vi "UI.vi"(0 "reference in":refnum<class "GUI NVM.lvclass">, 5 "error in (no error)":errorcluster) -> (14 "reference out":refnum<class "GUI NVM.lvclass">, 19 "error out":errorcluster)   [LabVIEW 2019, in "GUI NVM.lvclass"]
uses:
  GUI NVM.lvclass
  D:/GIT H4000/H4000/src/GUI_class/GUI.lvclass
  modbus engine custom/MB_ENGINE_class/Engine Alarms.ctl
  modbus engine custom/MB_ENGINE_class/Settings.ctl
  modbus engine custom/MB_ENGINE_class/cmd enum.ctl
  modbus engine custom/MB_ENGINE_class/Engine State.ctl
  GUI_class/GUI.lvclass/GUI.ctl
  TypeDef/Needle Valve Data.ctl
  TypeDef/Needle Valve State.ctl
  modbus engine custom/MB_ENGINE_class/Limits Status.ctl
  SV_Wrap/SharedVariableWrapper.lvclass/SharedVariableWrapper.ctl
  MessageAMC_class/MessageAMC.lvclass
  D:/GIT H4000/H4000/src/MessageInterface_class/MessageInterface.lvclass
  TypeDef/Needle Valve Settings.ctl
  0872259c-c1b7-4622-8eff-96544e628326.vi
  1b4fed76-272f-4eb9-b435-1b7916789d73.vi
  d0ca9bf2-7cd9-4c29-a03d-de1c10393a74.vi
  GUI_class/Set Win State.vi
  GUI_class/protected/GetSheredData.vi
  0872259c-c1b7-4622-8eff-96544e628326.vi/63923c93-3271-404a-8daf-727763f159bc.vi
  SV_Wrap/Write Var Info.vi
  SV_Wrap/Read Var Info.vi
  1b4fed76-272f-4eb9-b435-1b7916789d73.vi/fad6aa2d-1fd6-40e9-9208-cebdd25b163b.vi
  d0ca9bf2-7cd9-4c29-a03d-de1c10393a74.vi/ea186c4c-0445-4979-bfc0-5907181f2b8f.vi
  SV_Wrap/Read connection str.vi
  <userlib>/_OpenG.lib/time/time.llb/Tick Count (ms)__ogtk.vi
  GUI_class/GUI.lvclass
  MessageInterface_class/MessageInterface.lvclass
  SV_Wrap/SharedVariableWrapper.lvclass
  modbus engine custom/MB_ENGINE_class/MB_ENGINE.lvclass
panel:
  in  "Engine State":T1 items=["ACCELERATING", "DECELERATINGTOSTOP", "DECELERATING", "STEADY", "INDEX_ACCEL", "NDEX_RUN", "INDEX_DECEL", "INDEX_DWELL", "INACTIVE", "STANDBY", "STANDBYTOINACTIVE"]
  out "String 2":string
  out "String":string
  in  "clear fault":bool
  in  "stop":bool
  in  "close":bool
  in  "open":bool
  in  "Set_cmd":bool
  in  "cmd to write":T2 items=["0 Idle"=0, "1 GoTo Absolute Position"=1, "2 GoTo Relative"=2, "10 GoTo Home Position"=10, "11 Set Home Position"=11, "12 Set FindHome Mode"=12, "13 Reset FindHome Mode"=13, "14 Get FindHome State"=14, "20 Hard Stop"=20, "21 HiZ Stop"=21, "22 Soft Stop"=22, "30 Clear Fault"=30, "40 Encoder Set Home"=40, "70 Driver Init"=70]
  in  "set":bool
  out "Kinematic":T3
  out "Waveform Chart - Dark 3":dbl(graph) caption="Угол"
  out "encoder":i32(graph) caption="Энкодер"
  out "step":i32(graph) caption="ШАГ"
  out "Alarms":T4
  out "DO 19":bool
  out "Connect":bool
  in  "stop":bool
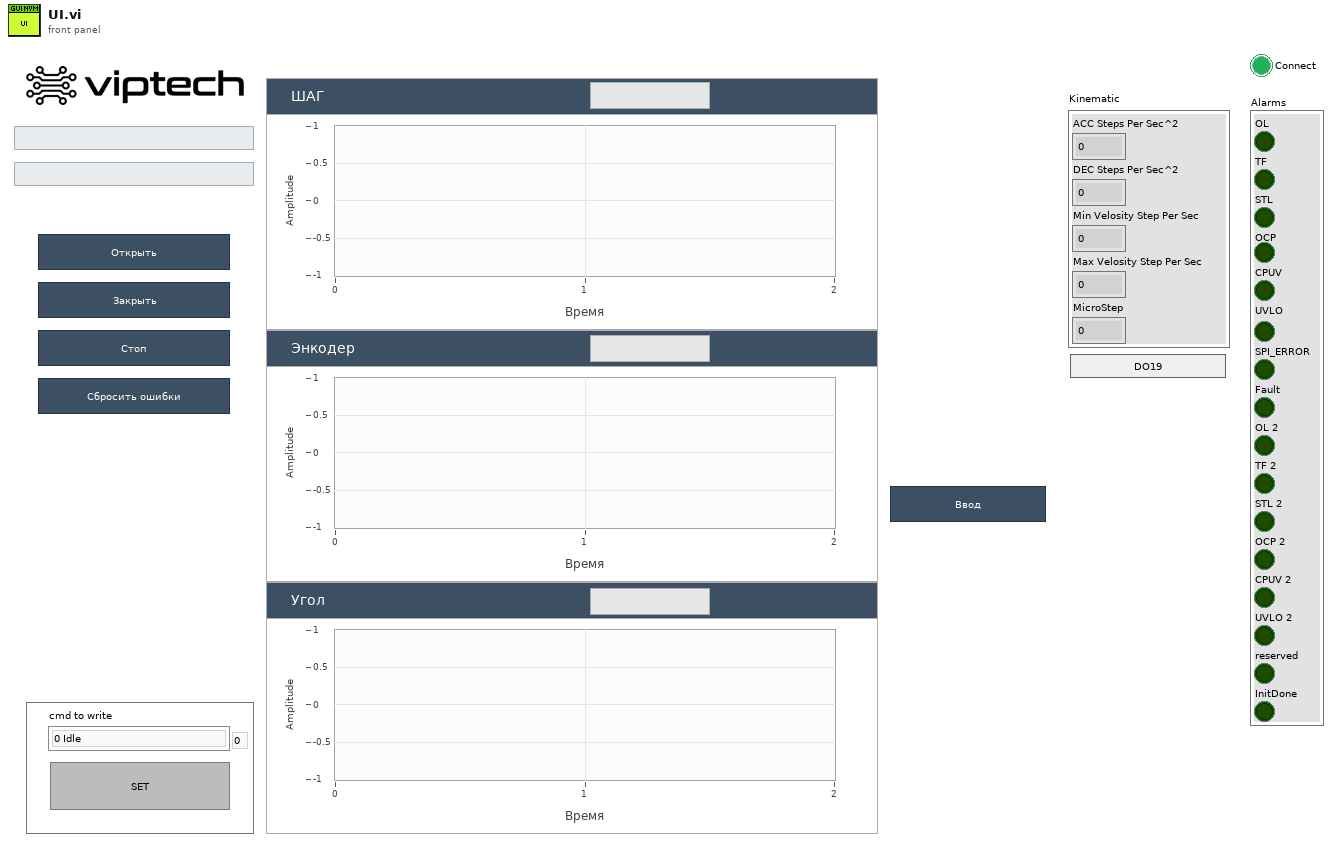
[diagram p1: front panel]
types:
  T1 = typedef "MB_ENGINE.lvclass/Engine State.ctl" = u16
  T2 = typedef "MB_ENGINE.lvclass/cmd enum.ctl" = u16
  T3 = typedef "MB_ENGINE.lvclass/Settings.ctl" = cluster{"ACC Steps Per Sec^2":u16, "DEC Steps Per Sec^2":u16, "Min Velosity Step Per Sec":u16, "Max Velosity Step Per Sec":u16, "MicroStep":u16}
  T4 = typedef "MB_ENGINE.lvclass/Engine Alarms.ctl" = cluster{"OL":bool, "TF":bool, "STL":bool, "OCP":bool, "CPUV":bool, "UVLO":bool, "SPI_ERROR":bool, "Fault":bool, "OL 2":bool, "TF 2":bool, "STL 2":bool, "OCP 2":bool, "CPUV 2":bool, "UVLO 2":bool, "reserved":bool, "InitDone":bool}
  T5 = enum32{"Invalid", "Standard", "Closed", "Hidden", "Minimized", "Maximized"}
  T6 = enum32{"invalid app kind", "Development System", "Run Time System", "Student Edition", "Embedded LabVIEW", "Evaluation", "Custom"}
  T7 = typedef "Needle Valve Settings.ctl" = cluster{"average size":i32, "open force":u16, "close force":u16, "open settings":T3, "close settings":T3}
  T8 = typedef "SharedVariableWrapper.lvclass/Config.ctl" = cluster{"connection str":string, "timeout":dbl, "ip":string}
  T9 = cluster{"Core":cluster{"Current VI Reference":refnum<vi>, "Close Panel on Exit?":bool}, "amc":refnum<class "MessageAMC.lvclass">, "settings_name_1":string}
  T10 = cluster{"Current VI Reference":refnum<vi>, "Close Panel on Exit?":bool}
  T11 = typedef "Needle Valve Data.ctl" = cluster{"Engine State":T1, "StateValveModbus":T12, "Alarms":T4, "RAW Possition":i32, "Angele":dbl, "Step":i32, "Encoder":i32, "Kinematic":T3, "Limits":T13}
  T12 = typedef "Needle Valve State.ctl" = enum16{"IDLE", "OPENING", "CLOSING", "STOP"}
  T13 = typedef "MB_ENGINE.lvclass/Limits Status.ctl" = cluster{"Fault 2 Switch":bool, "Fault 1 Switch":bool, "Center(Home)":bool, "Lower Limit":bool, "Upper Limit":bool}
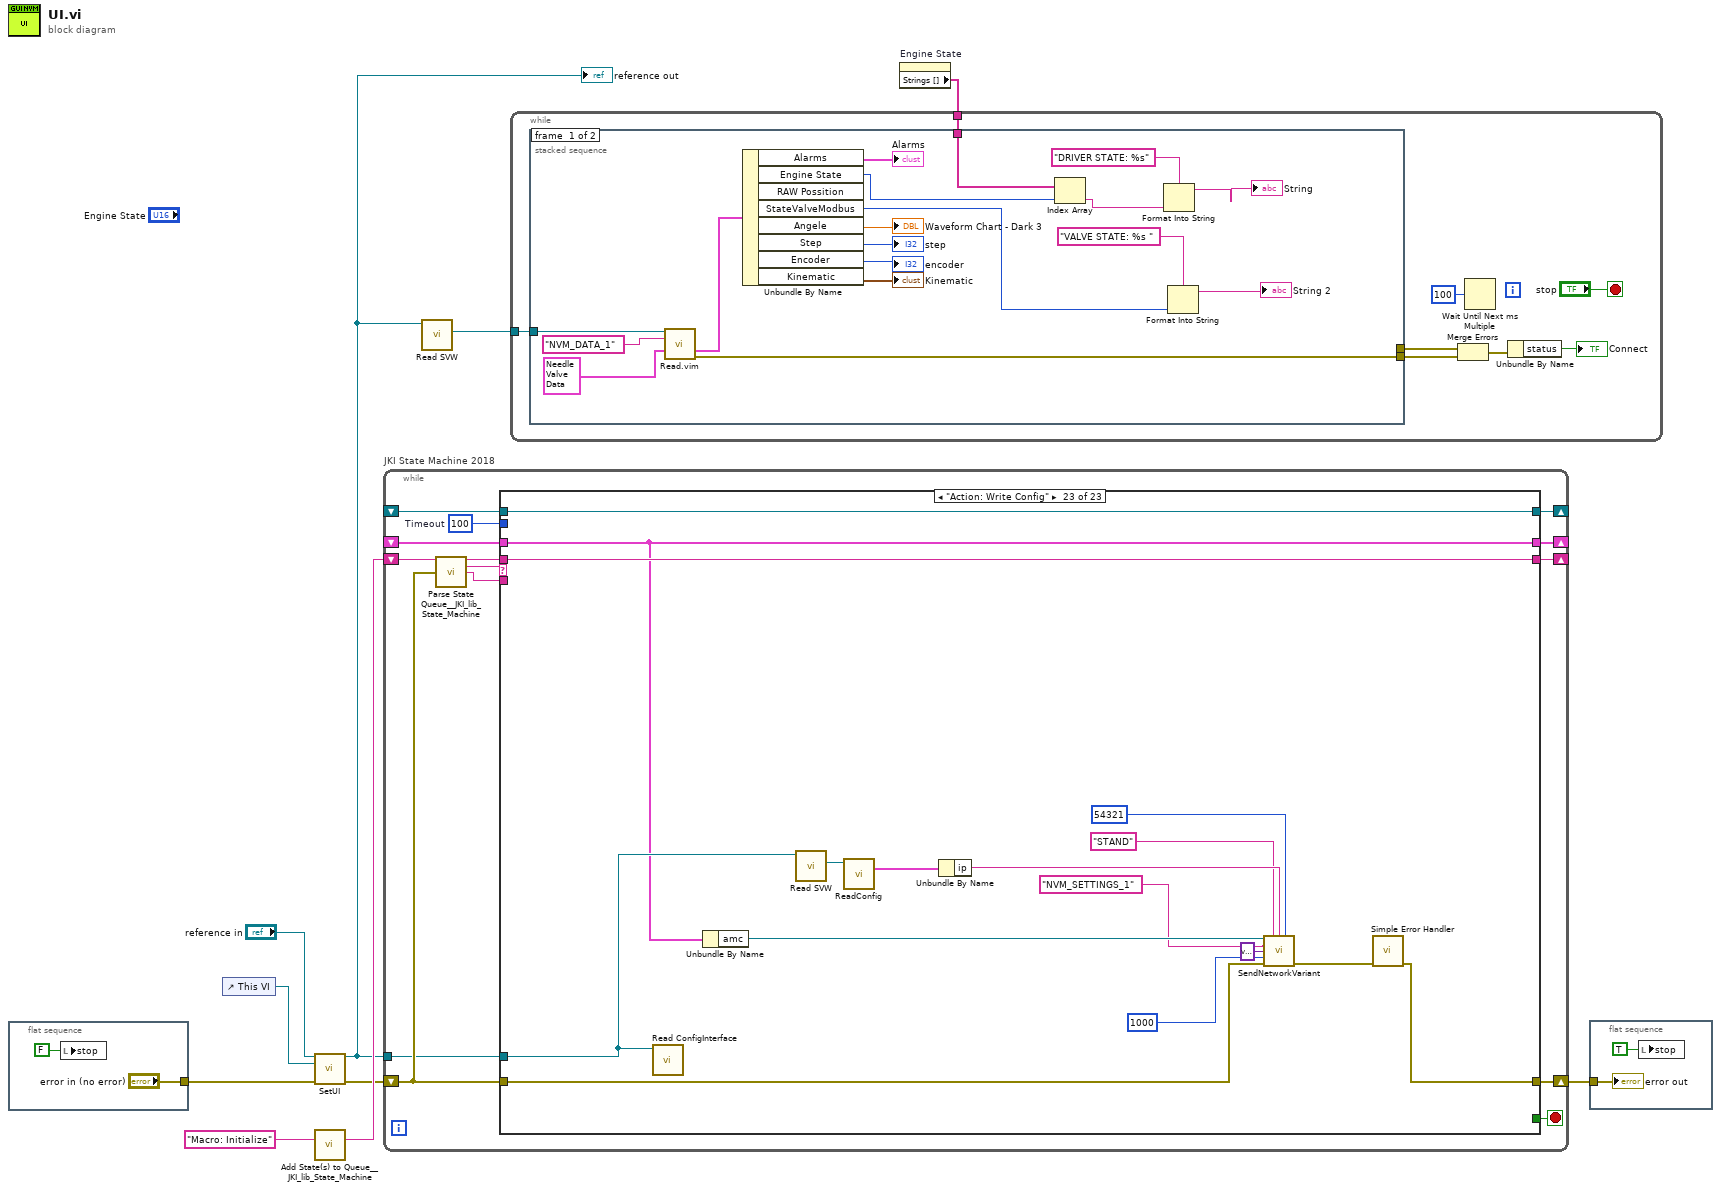
[diagram p0: block diagram]
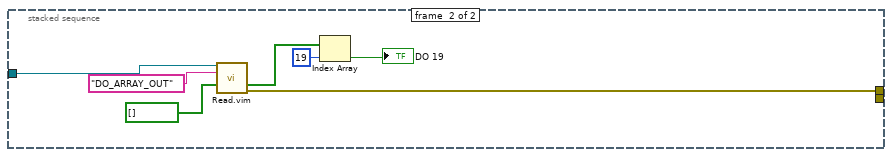
[diagram p2: hidden frame]
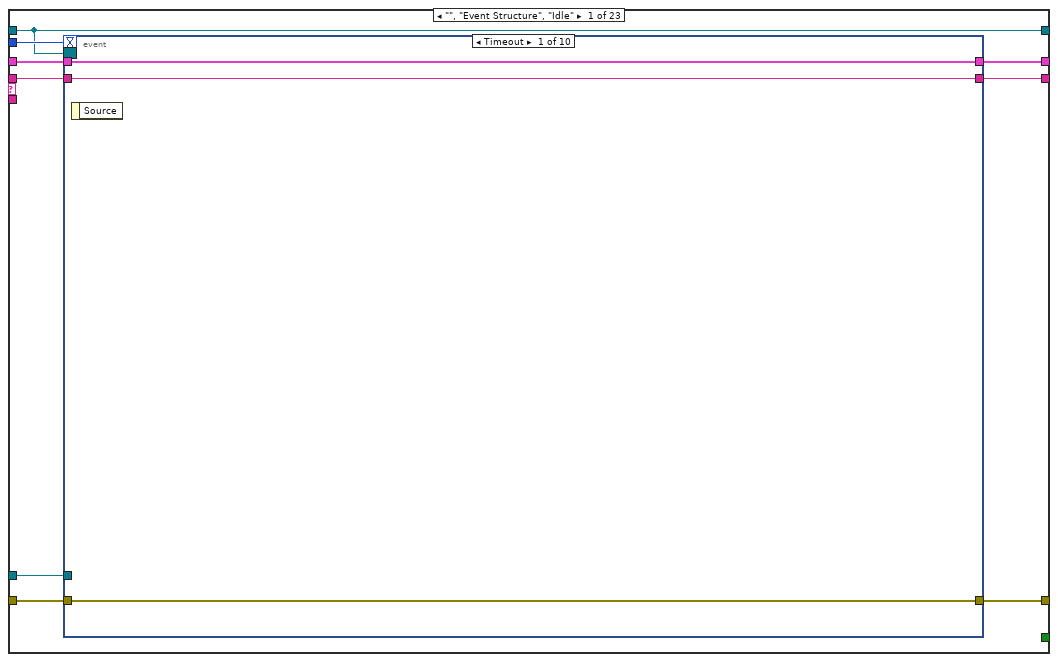
[diagram p3: hidden frame]
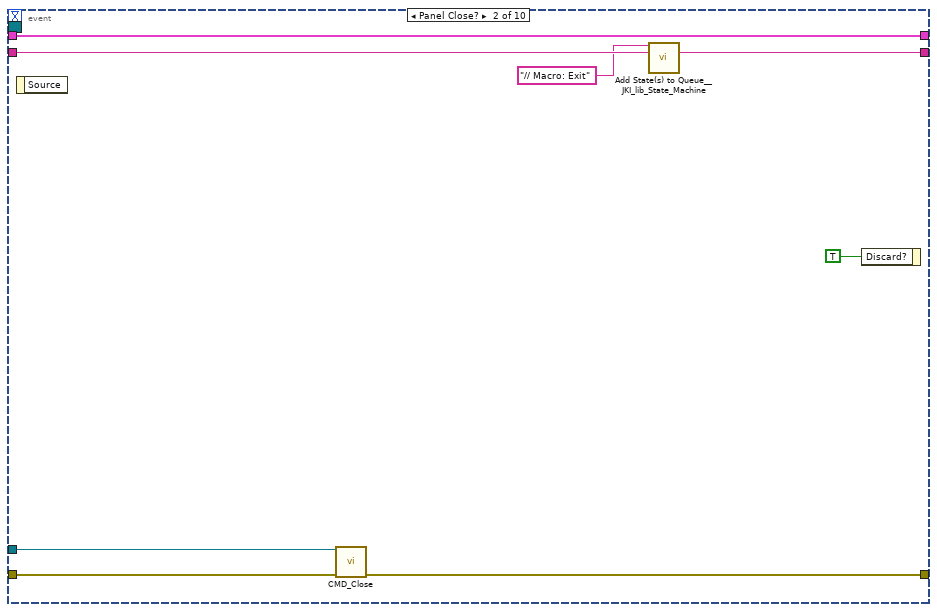
[diagram p4: hidden frame]
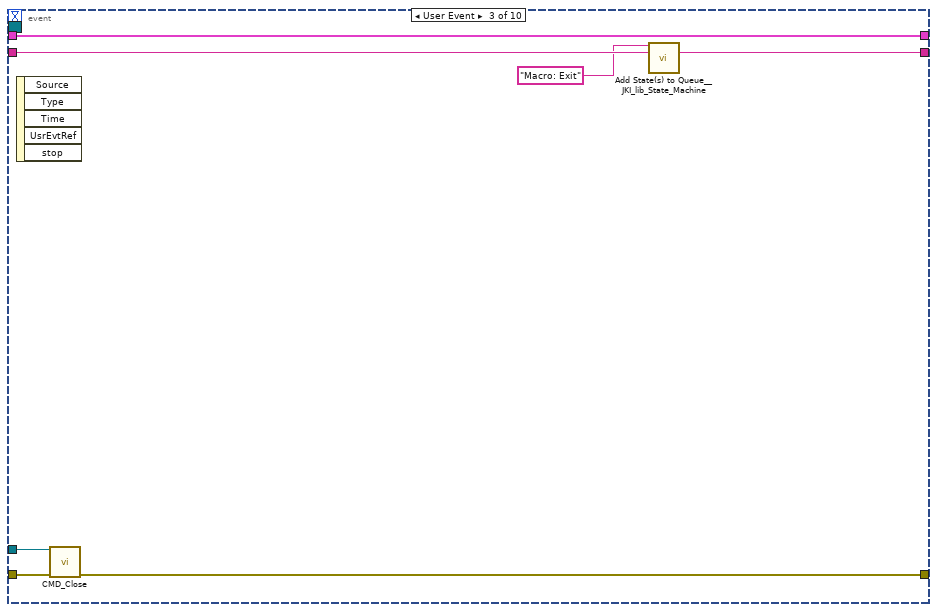
[diagram p5: hidden frame]
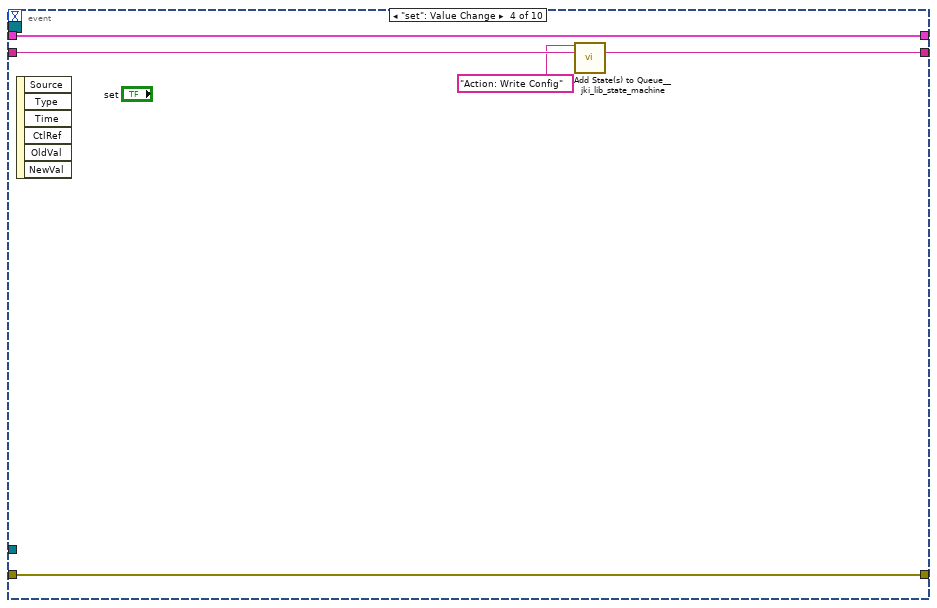
[diagram p6: hidden frame]
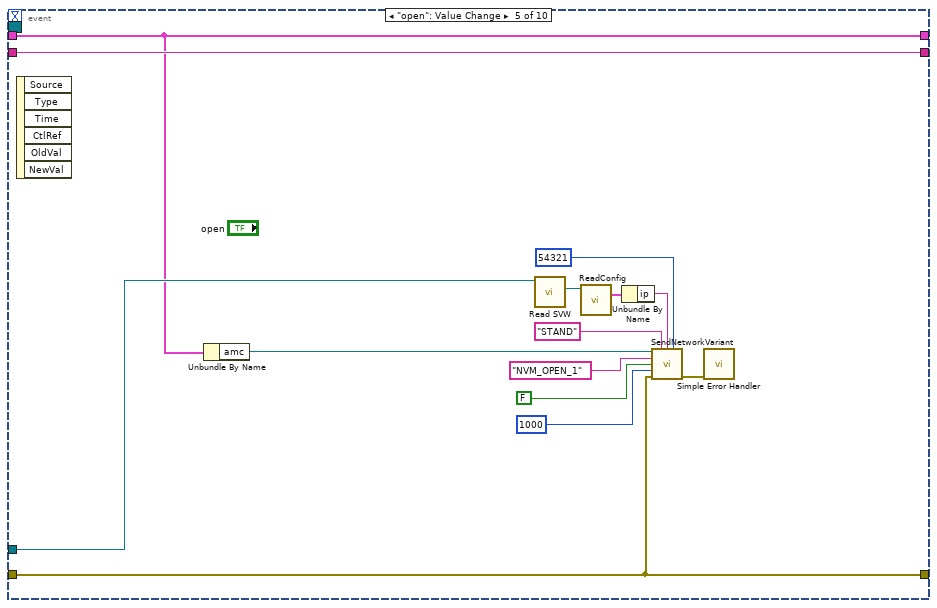
[diagram p7: hidden frame]
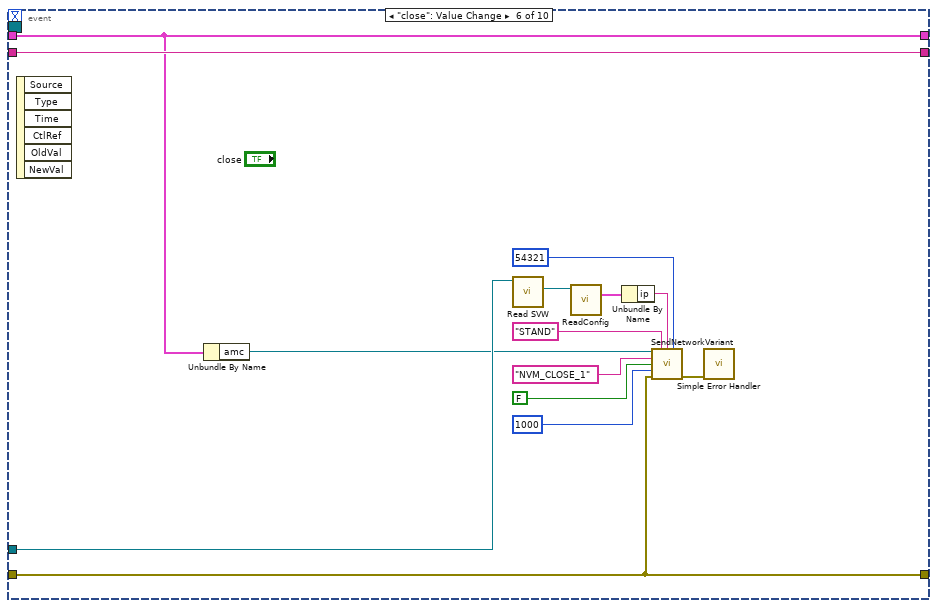
[diagram p8: hidden frame]
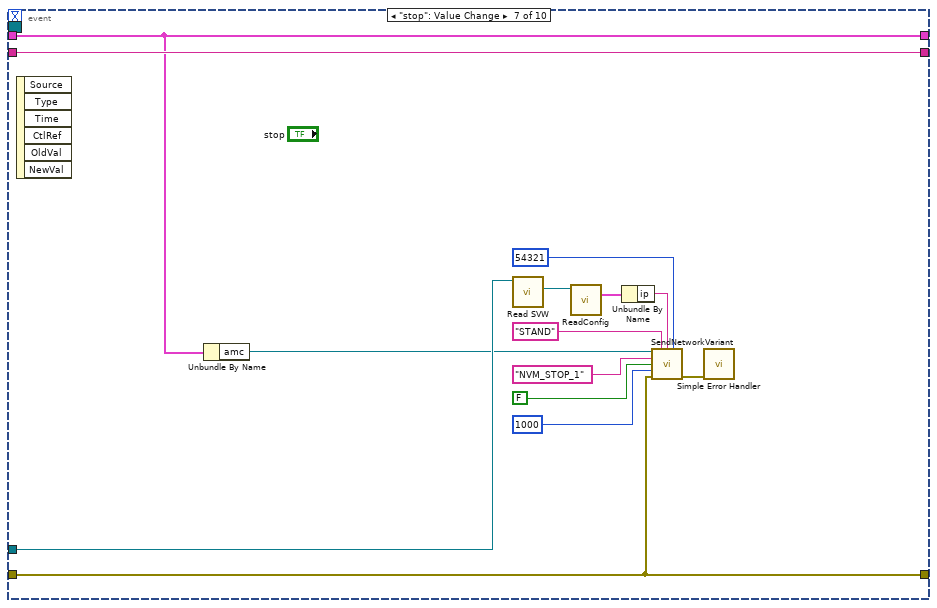
[diagram p9: hidden frame]
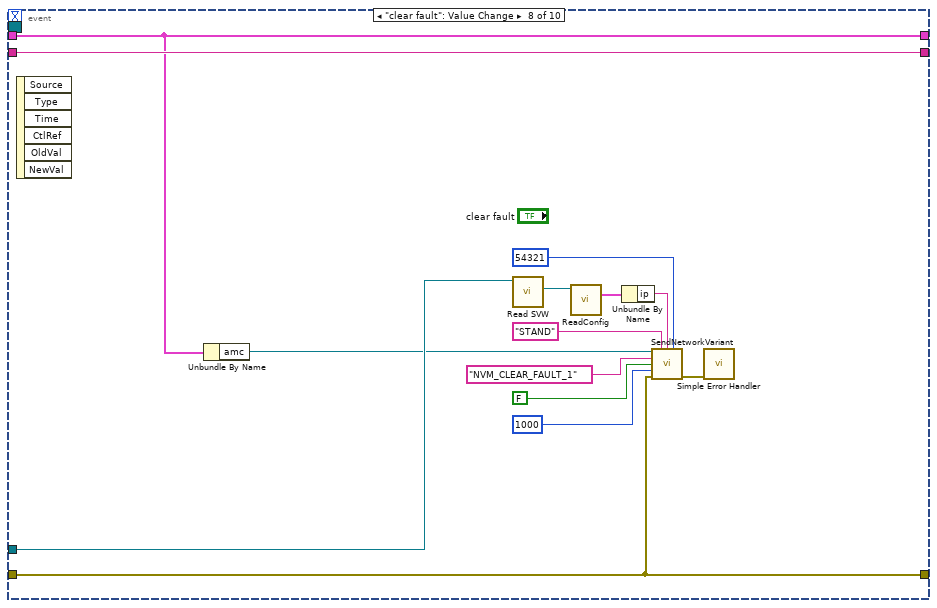
[diagram p10: hidden frame]
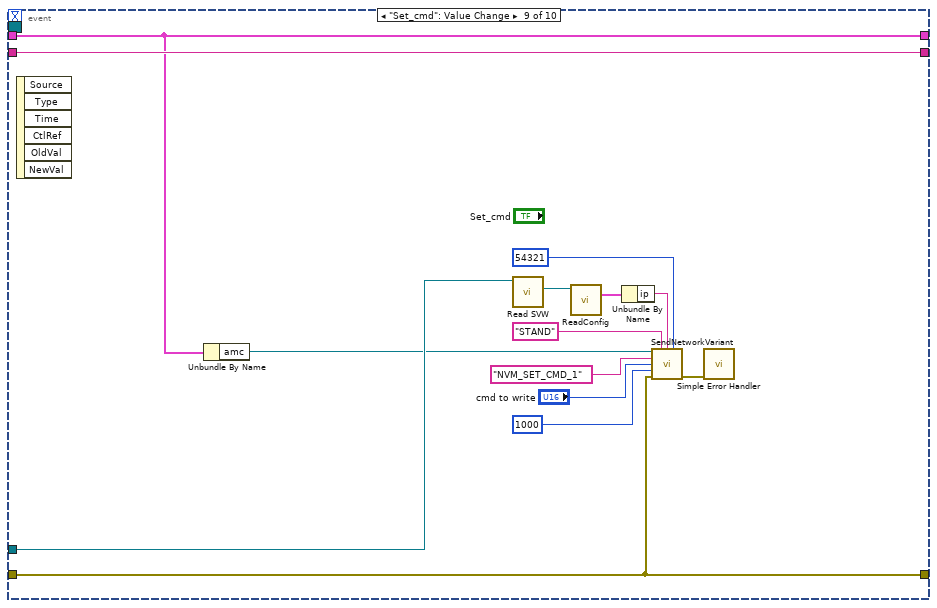
[diagram p11: hidden frame]
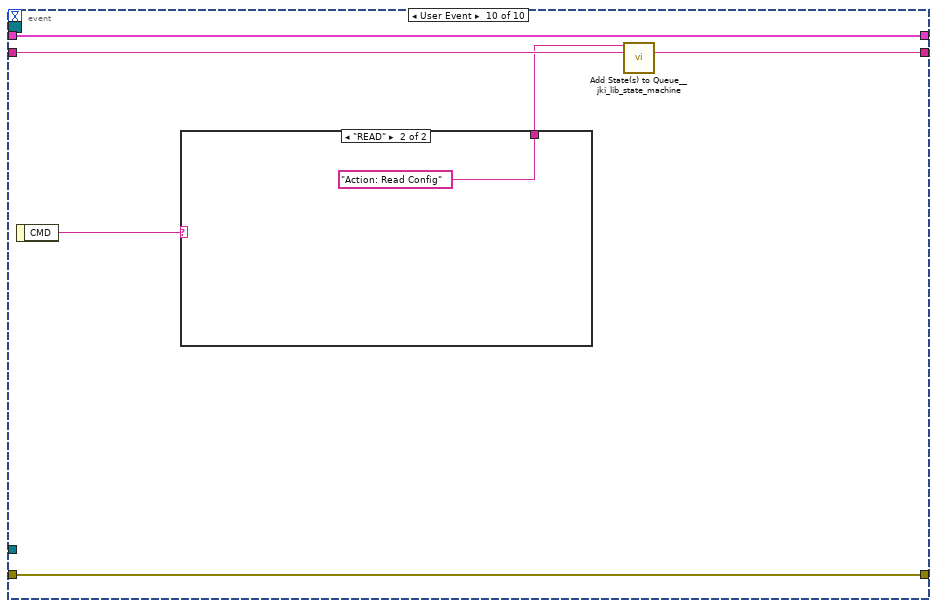
[diagram p12: hidden frame]
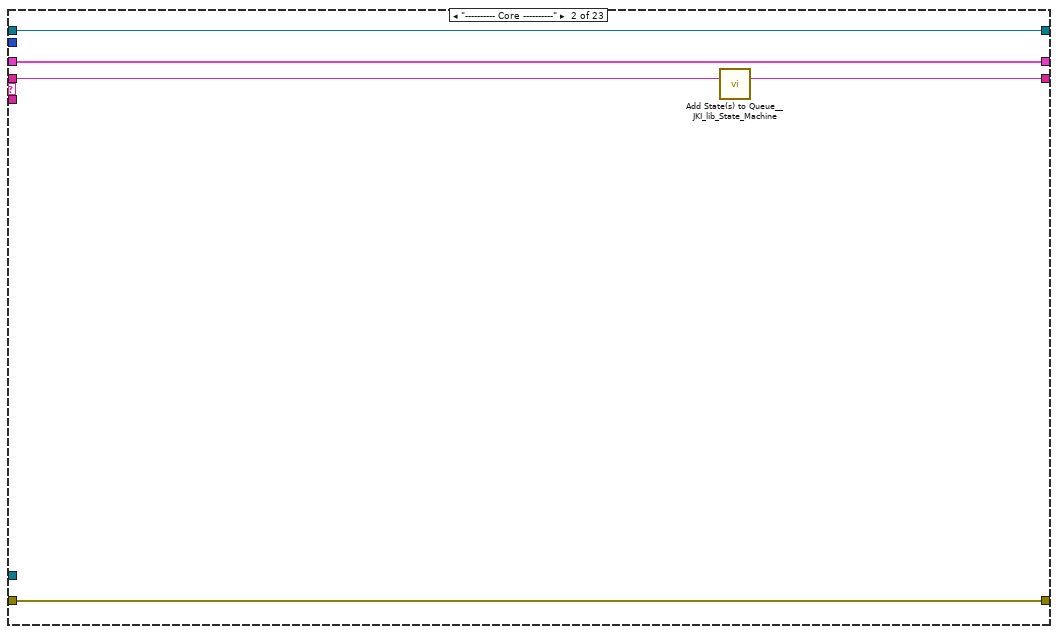
[diagram p14: hidden frame]
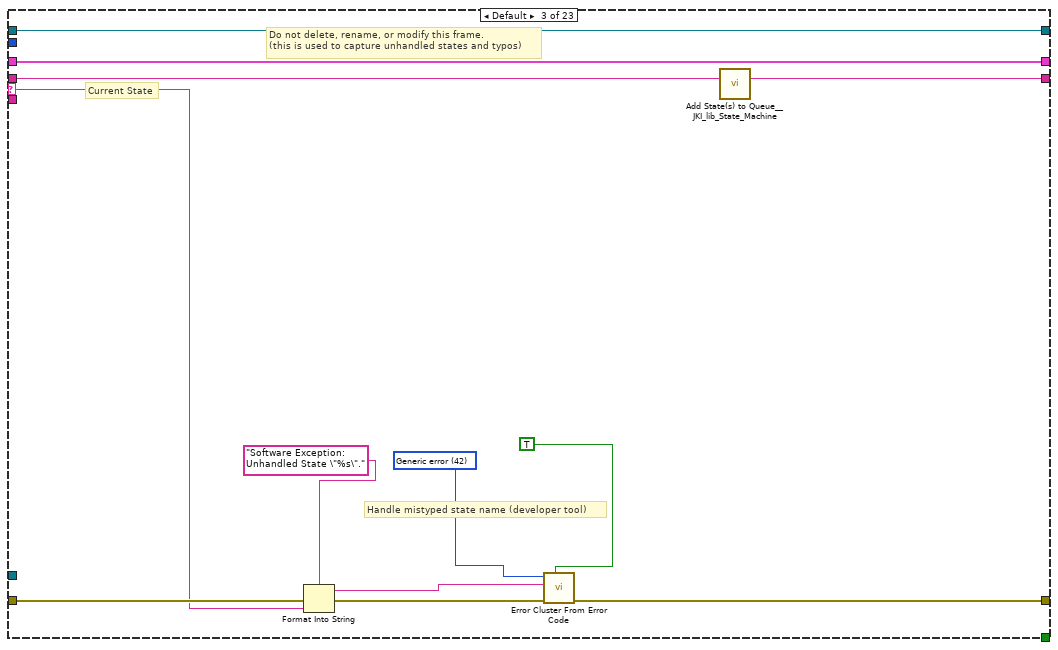
[diagram p15: hidden frame]
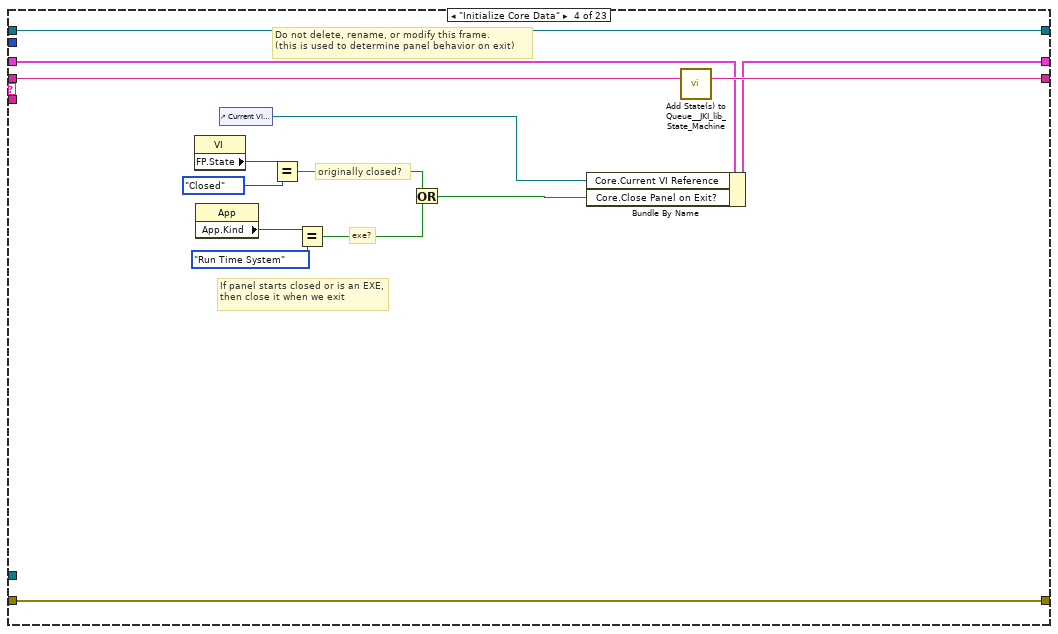
[diagram p16: hidden frame]
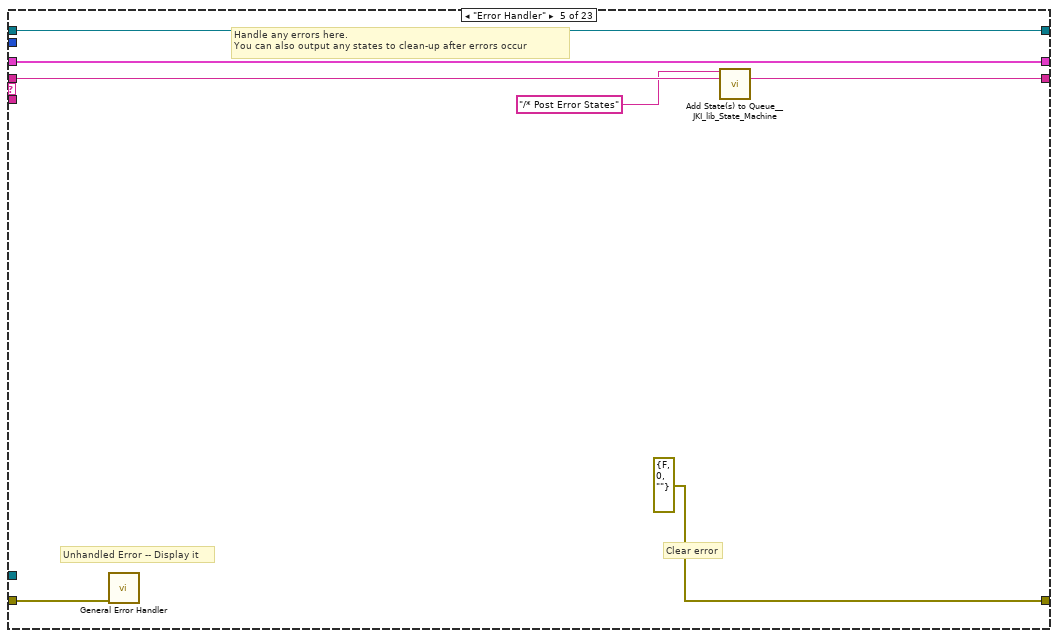
[diagram p17: hidden frame]
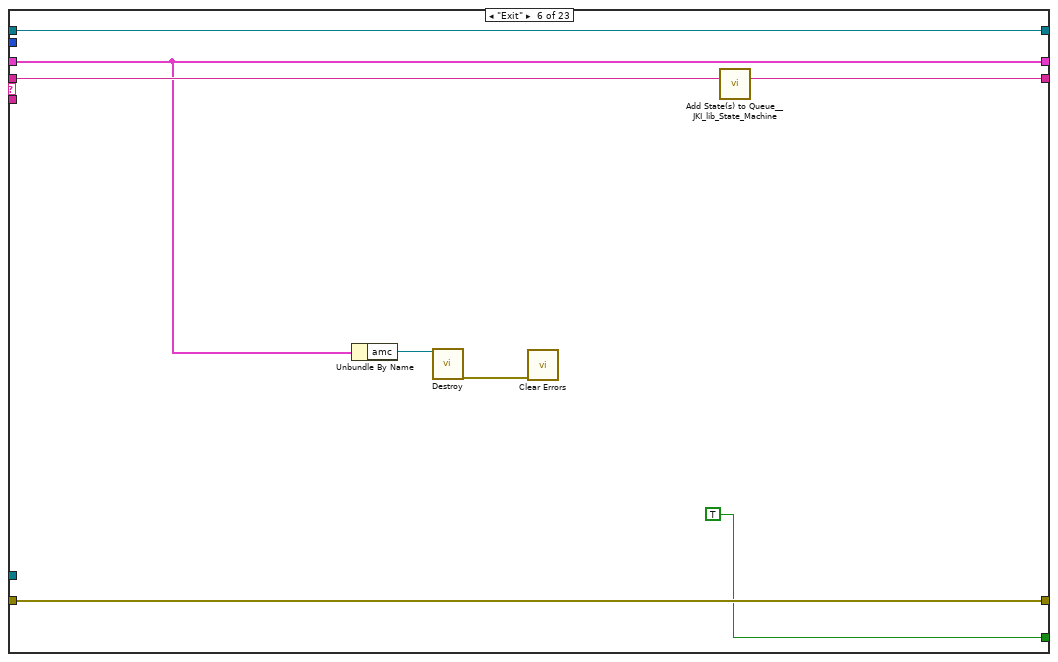
[diagram p18: hidden frame]
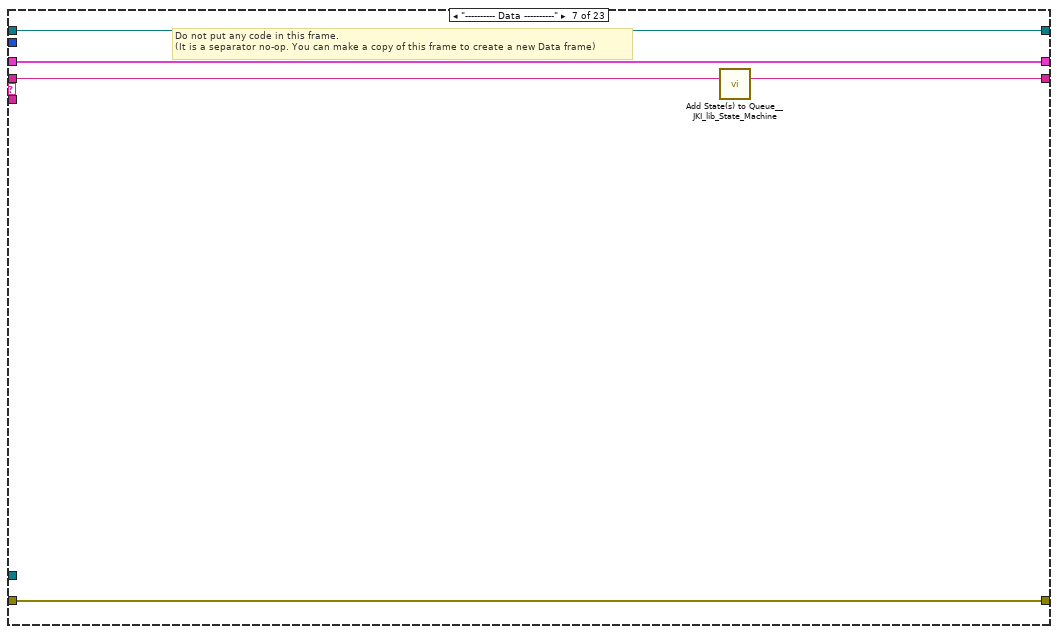
[diagram p19: hidden frame]
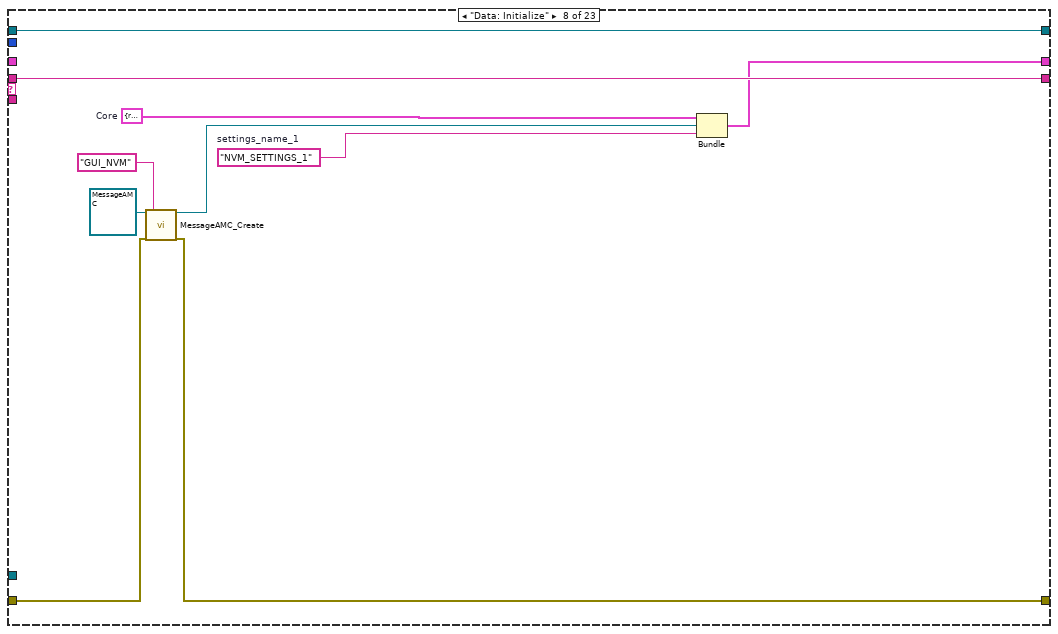
[diagram p20: hidden frame]
diagram:
  n1 = flat-sequence {
    tunnel: ["error in (no error)"] -> w7
    frame #0 {
      n2 = local write "stop"(FALSE ("stop")) -> ()
    }
  }
  n3 = control-ref of="This VI"() -> (w5:refnum<vi>)
  n4 = call "SetUI.vi"("reference in"="reference in", "UI VI"=w5, "error in (no error)"=w7) -> ("reference out"=w3:refnum<class "GUI NVM.lvclass">, "error out"=w4:errorcluster)  [unwired: 11 in]
  "reference out" <- w3
  n5 = call <vilib>:"Add State(s) to Queue__JKI_lib_State_Machine.vi"("State(s) in (\"\")"="Macro: Initialize") -> ("States Out"=w10:string)  [unwired: 14 in]
  n6 = while "JKI State Machine 2018" {
    shift-right: [w19] -> _
    shift-left: _ -> [w18]
    shift-right: [w22] -> w8
    shift-left: w4 -> [w16]
    shift-right: [w21] -> _
    shift-left: w10 -> [w23]
    tunnel: w3 -> [w15]
    shift-right: [w14] -> _
    shift-left: _ -> [w13]
    stop <- w20 stop-if-true
    w17 = 100  # Timeout
    n7 = call <vilib>:"Parse State Queue__JKI_lib_State_Machine.vi"("State Queue"=w23, "Error In (no error)"=w16) -> ("Remaining States"=w25:string, "Current State"=w26:string, "Arguments"=w24:string)  [unwired: 11 in]
    n8 = case shown="\"Action: Write Config\"" w26 {
      selector: w26 -> [_ _ w142 _ _ _ _ _ _ _ _ _ _ _ _ _ _ _ _ _ _ _ _]
      tunnel: w25 -> [w35 w140 w146 w166 w173 w181 w186 w196 w203 w208 w216 w222 w227 w231 w238 w250 w320 w326 w332 w344 w348 w351 w377]
      tunnel: w24 -> [_ _ _ _ _ _ _ _ _ _ _ _ _ _ w233 w244 _ _ _ _ _ _ _]
      tunnel: w18 -> [w33 w137 w144 w159 w170 w176 w183 _ w198 w205 w215 w220 w224 w230 w236 w246 w317 w323 w329 w341 w346 w353 w364]
      tunnel: [w32 w138 w148 w163 errorcluster {"status"=FALSE, "code"=0, "source"=""} ("error out") w179 w184 w189 w199 w206 w213 w217 w225 w229 w234 w247 w318 w324 w330 w342 w347 w354 w363] -> w22
      tunnel: w16 -> [w31 w138 w147 w163 w169 w179 w184 w190 w200 w206 w212 w218 w225 w229 w235 w248 w318 w324 w330 w342 w347 w355 w365]
      tunnel: [w34 w139 w145 w165 w172 w180 w185 w196 w202 w207 w216 w221 w226 w231 w237 w249 w319 w325 w331 w343 w348 w351 w377] -> w21
      tunnel: [_ _ _ _ _ TRUE _ _ _ _ _ _ _ _ _ _ _ _ _ _ _ _ _] -> w20
      tunnel: [w30 w137 w144 w164 w170 w176 w183 w195 w198 w205 w215 w220 w224 w230 w236 w246 w317 w323 w329 w341 w346 w352 w364] -> w19
      tunnel: w17 -> [w29 _ _ _ _ _ _ _ _ _ _ _ _ _ _ _ _ _ _ _ _ _ _]
      tunnel: w15 -> [w28 _ _ _ _ _ _ _ _ _ w211 _ _ _ _ _ _ _ _ _ _ w350 w366]
      tunnel: [w27 w136 w141 w153 w167 w177 w182 w193 w197 w204 w214 w219 w223 w228 w232 w243 w316 w321 w327 w334 w345 w356 w376] -> w14
      tunnel: w13 -> [w27 w136 w141 w153 w167 w177 w182 w193 w197 w204 _ w219 w223 w228 w232 w243 w316 w321 w327 w334 w345 w356 w376]
      frame "", "Event Structure", "Idle" {
        n9 = event shown="[0] Timeout" {
          selector: w27 -> [_ _ _ _ _ _ _ _ _ _]
          dyn-events: _ -> [_ _ _ _ _ _ _ _ _ _]
          timeout: w29 -> [_ _ _ _ _ _ _ _ _ _]
          tunnel: w35 -> [w38 w46 w53 w55 w72 w86 w100 w114 w128 w131]
          tunnel: [w38 w45 w52 w56 w72 w86 w100 w114 w128 w132] -> w34
          tunnel: w33 -> [w36 w44 w51 w57 w64 w78 w92 w106 w120 w133]
          tunnel: [w37 w39 w47 w58 w59 w73 w87 w101 w116 w134] -> w32
          tunnel: w31 -> [w37 w40 w48 w58 w59 w73 w87 w101 w116 w134]
          tunnel: [w36 w44 w51 w57 w64 w78 w92 w106 w120 w133] -> w30
          tunnel: w28 -> [_ w41 w49 _ w65 w79 w93 w107 w121 _]
          event Timeout {
            n10 = event-data() -> ()  [unwired: 1 in, 1 out]
          }
          event Panel Close? {
            n11 = event-data() -> ()  [unwired: 1 in, 1 out]
            n12 = call "CMD_Close.vi"("reference in"=w41, "error in (no error)"=w40) -> ("error out"=w39:errorcluster)  [unwired: 12 in, 1 out]
            n13 = call <vilib>:"Add State(s) to Queue__JKI_lib_State_Machine.vi"("State(s) in Front (\"\")"="// Macro: Exit", "State(s) in (\"\")"=w46) -> ("States Out"=w45:string)  [unwired: 13 in]
            n14 = event-data("Discard?"=TRUE) -> ()  [unwired: 1 in, 1 out]
          }
          event User Event {
            n15 = event-data() -> ()  [unwired: 1 in, 5 out]
            n16 = call "CMD_Close.vi"("reference in"=w49, "error in (no error)"=w48) -> ("error out"=w47:errorcluster)  [unwired: 12 in, 1 out]
            n17 = call <vilib>:"Add State(s) to Queue__JKI_lib_State_Machine.vi"("State(s) in Front (\"\")"="Macro: Exit", "State(s) in (\"\")"=w53) -> ("States Out"=w52:string)  [unwired: 13 in]
          }
          event "set": Value Change {
            n18 = event-data() -> ()  [unwired: 1 in, 6 out]
            n19 = call <vilib>:"Add State(s) to Queue__jki_lib_state_machine.vi"("State(s) in Front (\"\")"="Action: Write Config" ("State(s) in Front (\"\")"), "State(s) in (\"\")"=w55) -> ("States Out"=w56:string)  [unwired: 13 in]
          }
          event "open": Value Change {
            n20 = event-data() -> ()  [unwired: 1 in, 6 out]
            n21 = Unbundle By Name(w64) -> ("amc"=w63:refnum<class "MessageAMC.lvclass">)
            n22 = call "Read SVW.vi"("GUI in"=w65) -> ("SharedVariableWrapper.lvclass"=w67:refnum<class "SharedVariableWrapper.lvclass">)  [unwired: 10 in]
            n23 = call "ReadConfig.vi"("SharedVariableWrapper in"=w67) -> ("config"=w66:T8)  [unwired: 12 in, 2 out]
            n24 = Unbundle By Name(w66) -> ("ip"=w62:string)
            n25 = call "SendNetworkVariant.vi"("reference in"=w63, "receiver process"="STAND", "receiver host"=w62, "receiver port (0)"=u16 54321, "name"="NVM_OPEN_1", "data"=FALSE, "timeout (25000 ms)"=1000, "error in (no error)"=w59) -> ("error out"=w60:errorcluster)  [unwired: 5 in, 2 out]
            n26 = call <vilib>:"Simple Error Handler.vi"("error in (no error)"=w60) -> ()  [unwired: 4 in, 5 out]
          }
          event "close": Value Change {
            n27 = event-data() -> ()  [unwired: 1 in, 6 out]
            n28 = Unbundle By Name(w78) -> ("amc"=w77:refnum<class "MessageAMC.lvclass">)
            n29 = call "Read SVW.vi"("GUI in"=w79) -> ("SharedVariableWrapper.lvclass"=w81:refnum<class "SharedVariableWrapper.lvclass">)  [unwired: 10 in]
            n30 = call "ReadConfig.vi"("SharedVariableWrapper in"=w81) -> ("config"=w80:T8)  [unwired: 12 in, 2 out]
            n31 = Unbundle By Name(w80) -> ("ip"=w76:string)
            n32 = call "SendNetworkVariant.vi"("reference in"=w77, "receiver process"="STAND", "receiver host"=w76, "receiver port (0)"=u16 54321, "name"="NVM_CLOSE_1", "data"=FALSE, "timeout (25000 ms)"=1000, "error in (no error)"=w73) -> ("error out"=w74:errorcluster)  [unwired: 5 in, 2 out]
            n33 = call <vilib>:"Simple Error Handler.vi"("error in (no error)"=w74) -> ()  [unwired: 4 in, 5 out]
          }
          event "stop": Value Change {
            n34 = event-data() -> ()  [unwired: 1 in, 6 out]
            n35 = Unbundle By Name(w92) -> ("amc"=w91:refnum<class "MessageAMC.lvclass">)
            n36 = call "Read SVW.vi"("GUI in"=w93) -> ("SharedVariableWrapper.lvclass"=w95:refnum<class "SharedVariableWrapper.lvclass">)  [unwired: 10 in]
            n37 = call "ReadConfig.vi"("SharedVariableWrapper in"=w95) -> ("config"=w94:T8)  [unwired: 12 in, 2 out]
            n38 = Unbundle By Name(w94) -> ("ip"=w90:string)
            n39 = call "SendNetworkVariant.vi"("reference in"=w91, "receiver process"="STAND", "receiver host"=w90, "receiver port (0)"=u16 54321, "name"="NVM_STOP_1", "data"=FALSE, "timeout (25000 ms)"=1000, "error in (no error)"=w87) -> ("error out"=w88:errorcluster)  [unwired: 5 in, 2 out]
            n40 = call <vilib>:"Simple Error Handler.vi"("error in (no error)"=w88) -> ()  [unwired: 4 in, 5 out]
          }
          event "clear fault": Value Change {
            n41 = event-data() -> ()  [unwired: 1 in, 6 out]
            n42 = Unbundle By Name(w106) -> ("amc"=w105:refnum<class "MessageAMC.lvclass">)
            n43 = call "Read SVW.vi"("GUI in"=w107) -> ("SharedVariableWrapper.lvclass"=w109:refnum<class "SharedVariableWrapper.lvclass">)  [unwired: 10 in]
            n44 = call "ReadConfig.vi"("SharedVariableWrapper in"=w109) -> ("config"=w108:T8)  [unwired: 12 in, 2 out]
            n45 = Unbundle By Name(w108) -> ("ip"=w104:string)
            n46 = call "SendNetworkVariant.vi"("reference in"=w105, "receiver process"="STAND", "receiver host"=w104, "receiver port (0)"=u16 54321, "name"="NVM_CLEAR_FAULT_1", "data"=FALSE, "timeout (25000 ms)"=1000, "error in (no error)"=w101) -> ("error out"=w102:errorcluster)  [unwired: 5 in, 2 out]
            n47 = call <vilib>:"Simple Error Handler.vi"("error in (no error)"=w102) -> ()  [unwired: 4 in, 5 out]
          }
          event "Set_cmd": Value Change {
            n48 = event-data() -> ()  [unwired: 1 in, 6 out]
            n49 = Unbundle By Name(w120) -> ("amc"=w119:refnum<class "MessageAMC.lvclass">)
            n50 = call "Read SVW.vi"("GUI in"=w121) -> ("SharedVariableWrapper.lvclass"=w123:refnum<class "SharedVariableWrapper.lvclass">)  [unwired: 10 in]
            n51 = call "ReadConfig.vi"("SharedVariableWrapper in"=w123) -> ("config"=w122:T8)  [unwired: 12 in, 2 out]
            n52 = Unbundle By Name(w122) -> ("ip"=w118:string)
            n53 = call "SendNetworkVariant.vi"("reference in"=w119, "receiver process"="STAND", "receiver host"=w118, "receiver port (0)"=u16 54321, "name"="NVM_SET_CMD_1", "data"="cmd to write", "timeout (25000 ms)"=1000, "error in (no error)"=w116) -> ("error out"=w117:errorcluster)  [unwired: 5 in, 2 out]
            n54 = call <vilib>:"Simple Error Handler.vi"("error in (no error)"=w117) -> ()  [unwired: 4 in, 5 out]
          }
          event User Event {
            n55 = event-data() -> ("CMD"=w130:string)  [unwired: 1 in]
            n56 = case shown="\"READ\"" w130 {
              tunnel: [_ "Action: Read Config" ("State(s) in Front (\"\")")] -> w129
              frame "False", Default {
              }
              frame "READ" {
              }
            }
            n57 = call <vilib>:"Add State(s) to Queue__jki_lib_state_machine.vi"("State(s) in Front (\"\")"=w129, "State(s) in (\"\")"=w131) -> ("States Out"=w132:string)  [unwired: 13 in]
          }
        }
      }
      frame "---------- Core ----------" {
        n58 = call <vilib>:"Add State(s) to Queue__JKI_lib_State_Machine.vi"("State(s) in (\"\")"=w140) -> ("States Out"=w139:string)  [unwired: 14 in]
      }
      frame Default {
        w151 = 42 items=["No error", "Argument error", "Memory is full", "Out of zone", "End of file", "File already open", "Generic file I/O error", "File not found", "File permission error", "Disk is full", "Duplicate path", "Too many files open", "System feature not enabled", "Resource file not found", "Cannot add resource", "Resource not found", "Image not found", "Image memory error", "Pen does not exist", "Config type invalid", "Config token not found", "Config parse error", "Config memory error", "Bad external code format", "Bad external code offset", "External code not present", "Null window", "Destroy window error", "Null menu", "Print aborted", "Bad print record", "Print driver error", "Windows error during printing", "Memory error during printing", "Print dialog error", "Generic print error", "Invalid device refnum", "Device not found", "Device parameter error", "Device unit error", "Cannot open device", "Device call aborted", "Generic error", "Cancelled by user", "Object ID too low", "Object ID too high", "Object not in heap", "Unknown heap", "Unknown object (invalid DefProc)", "Unknown object (DefProc not in table)", "Message out of range", "Invalid (null) method", "Unknown message", "Manager call not supported", "Bad address", "Network operation in progress", "Network operation timed out", "Connection is busy", "Network attribute not supported", "Network error", "Address in use", "System out of memory", "Connection aborted", "Connection refused", "Not connected", "Already connected", "Connection closed", "Initialization error (interapplication manager)", "Bad occurrence", "Wait on unbound occurrence handler", "Occurrence queue overflow", "Datalog type conflict", "Unused", "Unrecognized type (interapplication manager)", "Memory corrupt", "Failed to make temporary DLL", "Old CIN version", "Drag socket not found", "Failed to load drop-object", "Failed to register OLE object", "Failed to release OLE object", "Format specifier type mismatch", "Unknown format specifier", "Too few format specifiers", "Too many format specifiers", "Scan failed", "Newer CIN version", "Error converting to variant", "Runtime menu error", "Password tampered", "Variant attribute not found", "Incompatible variant data type", "Event data is not available", "Event Store is not present", "Occurrence is not found", "Event Queue is not created", "Event info is not available", "Refnum passed is NULL", "Error retrieving Class GUID", "Error retrieving CoClass GUID", "Error retrieving TypeLib GUID.", "Bad built application magic bytes.", "Specific driver is different from the specific driver associated with the Logical Name.", "There is no session opened to the class driver.", "Max Error", "MAX - Error with config objects", "MAX - Error loading configuration", "MAX - Group not supported"]
        # "Current State"
        # "Do not delete, rename, or modify this frame.\n(this is used to capture unhandled states and typos)"
        # "Handle mistyped state name (developer tool)"
        n59 = Format Into String(format string="Software Exception: Unhandled State \"%s\"." ("message"), error in=w147, w142) -> (resulting string=w150:string, error out=w149:errorcluster)  [unwired: 1 in]
        n60 = call <vilib>:"Error Cluster From Error Code.vi"("show call chain? (False)"=TRUE, "error in (no error)"=w149, "error message (\"\")"=w150, "error code (0)"=w151) -> ("error out"=w148:errorcluster)  [unwired: 5 in]
        n61 = call <vilib>:"Add State(s) to Queue__JKI_lib_State_Machine.vi"("State(s) in (\"\")"=w146) -> ("States Out"=w145:string)  [unwired: 14 in]
      }
      frame "Initialize Core Data" {
        # "Do not delete, rename, or modify this frame.\n(this is used to determine panel behavior on exit)"
        # "originally closed?"
        # "exe?"
        # "If panel starts closed or is an EXE, then close it when we exit"
        n62 = property class="VI"() -> ("FP.State"=w156:T5)  [unwired: 2 in, 2 out]
        n63 = property class="App"() -> ("App.Kind"=w162:T6)  [unwired: 2 in, 2 out]
        n64 = control-ref of="Current VI Reference"() -> (w157:refnum<vi>)
        n65 = Equal?(x=w156, y=T5."Closed" ("Front Panel Window:State")) -> (x = y?=w154:bool)
        n66 = Equal?(x=w162, y=T6."Run Time System" ("Application:Kind")) -> (x = y?=w160:bool)
        n67 = Or(x=w154, y=w160) -> (x .or. y?=w158:bool)
        n68 = Bundle By Name(cluster=w159, "Core.Current VI Reference"=w157, "Core.Close Panel on Exit?"=w158) -> (w164:T9)
        n69 = call <vilib>:"Add State(s) to Queue__JKI_lib_State_Machine.vi"("State(s) in (\"\")"=w166) -> ("States Out"=w165:string)  [unwired: 14 in]
      }
      frame "Error Handler" {
        # "Unhandled Error -- Display it"
        # "Handle any errors here.\nYou can also output any states to clean-up after errors occur"
        # "Clear error"
        n70 = call <vilib>:"General Error Handler.vi"("error in (no error)"=w169) -> ()  [unwired: 10 in, 5 out]
        n71 = call <vilib>:"Add State(s) to Queue__JKI_lib_State_Machine.vi"("State(s) in Front (\"\")"="/* Post Error States", "State(s) in (\"\")"=w173) -> ("States Out"=w172:string)  [unwired: 13 in]
      }
      frame "Exit" {
        n72 = Unbundle By Name(w176) -> ("amc"=w175:refnum<class "MessageAMC.lvclass">)
        n73 = call-dynamic "Destroy.vi"("reference in"=w175) -> ("error out"=w174:errorcluster)  [unwired: 17 in, 1 out]
        n74 = call <vilib>:"Clear Errors.vi"("error in (no error)"=w174) -> ()  [unwired: 5 in, 2 out]
        n75 = call <vilib>:"Add State(s) to Queue__JKI_lib_State_Machine.vi"("State(s) in (\"\")"=w181) -> ("States Out"=w180:string)  [unwired: 14 in]
      }
      frame "---------- Data ----------" {
        # "Do not put any code in this frame.\n(It is a separator no-op. You can make a copy of this frame to create a new Data frame)"
        n76 = call <vilib>:"Add State(s) to Queue__JKI_lib_State_Machine.vi"("State(s) in (\"\")"=w186) -> ("States Out"=w185:string)  [unwired: 14 in]
      }
      frame "Data: Initialize" {
        w187 = "NVM_SETTINGS_1"  # settings_name_1
        w194 = T10 {"Current VI Reference"=refnum, "Close Panel on Exit?"=FALSE}  # Core
        n77 = call "MessageAMC_Create.vi"("reference in"=refnum<class "MessageAMC.lvclass"> refnum, "error in (no error)"=w190, "message queue name"="GUI_NVM") -> ("amc"=w191:refnum<class "MessageAMC.lvclass">, "error out"=w189:errorcluster)  [unwired: 15 in]
        n78 = Bundle("Core"=w194, "amc"=w191, "settings_name_1"=w187) -> (w195:T9)  [unwired: 1 in]
      }
      frame "Data: Cleanup" {
        # "Cleanup any data and references, here.\n(this is called automatically, by the Macro: Exit)"
        n79 = Unbundle By Name(w198) -> ("Core.Current VI Reference"=w201:refnum<vi>)
        n80 = Close Reference(reference=w201, error in (no error)=w200) -> (error out=w199:errorcluster)
        n81 = call <vilib>:"Add State(s) to Queue__JKI_lib_State_Machine.vi"("State(s) in (\"\")"=w203) -> ("States Out"=w202:string)  [unwired: 14 in]
      }
      frame "---------- Events ----------" {
        # "Do not put any code in this frame.\n(It is a separator no-op. You can make a copy of this frame to create a new UI frame)"
        n82 = call <vilib>:"Add State(s) to Queue__JKI_lib_State_Machine.vi"("State(s) in (\"\")"=w208) -> ("States Out"=w207:string)  [unwired: 14 in]
      }
      frame "Events: Register" {
        n83 = call "Read stop event.vi"("GUI in"=w211) -> ("cmd event"=w209:refnum<user-event>, "stop event"=w210:refnum<user-event>)  [unwired: 8 in, 1 out]
        n84 = register-events(error in=w212, w210, w209) -> (reference out=w214:refnum<event-registration>, error out=w213:errorcluster)  [unwired: 1 in]
      }
      frame "Events: Unregister" {
        # "Do not put any code in this frame.\n(It is a separator no-op. You can make a copy of this frame to create a new UI frame)"
        n85 = Unregister For Events(event registration refnum=w219, error in=w218) -> (error out=w217:errorcluster)
        n86 = call <vilib>:"Add State(s) to Queue__JKI_lib_State_Machine.vi"("State(s) in (\"\")"=w222) -> ("States Out"=w221:string)  [unwired: 14 in]
      }
      frame "---------- UI ----------" {
        # "Do not put any code in this frame.\n(It is a separator no-op. You can make a copy of this frame to create a new UI frame)"
        n87 = call <vilib>:"Add State(s) to Queue__JKI_lib_State_Machine.vi"("State(s) in (\"\")"=w227) -> ("States Out"=w226:string)  [unwired: 14 in]
      }
      frame "UI: Initialize" {
      }
      frame "UI: Cursor Set" {
        # "Argument"
        # "Set and Unset Cursor Busy.\n(Usage: \"UI: Cursor Set >> Busy|Idle\")"
        n88 = case shown="\"Idle\", Default" w233 {
          tunnel: w235 -> [w240 w242]
          tunnel: [w239 w241] -> w234
          frame "Idle", Default {
            n89 = call <vilib>:"Unset Busy.vi"("error in (no error)"=w240) -> ("error out"=w239:errorcluster)  [unwired: 10 in]
          }
          frame "Busy" {
            n90 = call <vilib>:"Set Busy.vi"("error in (no error)"=w242) -> ("error out"=w241:errorcluster)  [unwired: 9 in, 1 out]
          }
        }
        n91 = call <vilib>:"Add State(s) to Queue__JKI_lib_State_Machine.vi"("State(s) in (\"\")"=w238) -> ("States Out"=w237:string)  [unwired: 14 in]
      }
      frame "UI: Front Panel State" {
        # "Argument"
        # "Set Front Panel Open or Closed\n(Usage: \"UI: Front Panel State >> Open|Close\")"
        n92 = Unbundle By Name(w246) -> ("Core.Current VI Reference"=w245:refnum<vi>)
        n93 = case shown="\"Minimize\", \"Minimized\"" w244 {
          tunnel: w248 -> [w256 w271 w282 w295 w308]
          tunnel: [w258 w272 w284 w297 w310] -> w247
          tunnel: w245 -> [w257 w269 w283 w296 w309]
          frame "Open", "Standard", Default {
            w251 = T5."Standard" ("State")
            n94 = property class="VI"(reference=w257, error in=w256) -> (reference out=w254:refnum<vi>, error out=w255:errorcluster, "FP.State"=w253:T5)
            n95 = Not Equal?(x=w253, y=w251) -> (x != y?=w252:bool)
            n96 = case shown="True" w252 {
              tunnel: [w262 w264] -> w258
              tunnel: w255 -> [w261 w264]
              tunnel: w254 -> [w260 _]
              tunnel: w251 -> [w259 _]
              frame True {
                n97 = invoke class="VI" method="FP.Open"(reference=w260, error in=w261, "Activate"=TRUE, "State"=w259) -> (error out=w262:errorcluster)  [unwired: 1 in, 4 out]
              }
              frame False {
              }
            }
          }
          frame "Close", "Closed" {
            n98 = property class="VI"(reference=w269, error in=w271) -> (reference out=w268:refnum<vi>, error out=w270:errorcluster, "FP.State"=w266:T5)
            n99 = Not Equal?(x=w266, y=T5."Closed" ("Front Panel Window:State")) -> (x != y?=w265:bool)
            n100 = case shown="True" w265 {
              tunnel: [w273 w276] -> w272
              tunnel: w270 -> [w273 w275]
              tunnel: w268 -> [_ w274]
              frame False {
              }
              frame True {
                n101 = invoke class="VI" method="FP.Close"(reference=w274, error in=w275) -> (error out=w276:errorcluster)  [unwired: 1 in, 2 out]
              }
            }
          }
          frame "Hidden", "Hide" {
            w277 = T5."Hidden" ("State")
            n102 = property class="VI"(reference=w283, error in=w282) -> (reference out=w280:refnum<vi>, error out=w281:errorcluster, "FP.State"=w279:T5)
            n103 = Not Equal?(x=w279, y=w277) -> (x != y?=w278:bool)
            n104 = case shown="True" w278 {
              tunnel: [w288 w289] -> w284
              tunnel: w281 -> [w287 w289]
              tunnel: w280 -> [w286 _]
              tunnel: w277 -> [w285 _]
              frame True {
                n105 = invoke class="VI" method="FP.Open"(reference=w286, error in=w287, "State"=w285) -> (error out=w288:errorcluster)  [unwired: 2 in, 4 out]
              }
              frame False {
              }
            }
          }
          frame "Minimize", "Minimized" {
            w290 = T5."Minimized" ("State")
            n106 = property class="VI"(reference=w296, error in=w295) -> (reference out=w293:refnum<vi>, error out=w294:errorcluster, "FP.State"=w292:T5)
            n107 = Not Equal?(x=w292, y=w290) -> (x != y?=w291:bool)
            n108 = case shown="True" w291 {
              tunnel: [w301 w302] -> w297
              tunnel: w294 -> [w300 w302]
              tunnel: w293 -> [w299 _]
              tunnel: w290 -> [w298 _]
              frame True {
                n109 = invoke class="VI" method="FP.Open"(reference=w299, error in=w300, "State"=w298) -> (error out=w301:errorcluster)  [unwired: 2 in, 4 out]
              }
              frame False {
              }
            }
          }
          frame "Maximize", "Maximized" {
            w303 = T5."Maximized" ("State")
            n110 = property class="VI"(reference=w309, error in=w308) -> (reference out=w306:refnum<vi>, error out=w307:errorcluster, "FP.State"=w305:T5)
            n111 = Not Equal?(x=w305, y=w303) -> (x != y?=w304:bool)
            n112 = case shown="True" w304 {
              tunnel: [w314 w315] -> w310
              tunnel: w307 -> [w313 w315]
              tunnel: w306 -> [w312 _]
              tunnel: w303 -> [w311 _]
              frame True {
                n113 = invoke class="VI" method="FP.Open"(reference=w312, error in=w313, "State"=w311) -> (error out=w314:errorcluster)  [unwired: 2 in, 4 out]
              }
              frame False {
              }
            }
          }
        }
        n114 = call <vilib>:"Add State(s) to Queue__JKI_lib_State_Machine.vi"("State(s) in (\"\")"=w250) -> ("States Out"=w249:string)  [unwired: 14 in]
      }
      frame "---------- Macro ----------" {
        # "Do not put any code in this frame.\n(It is a separator no-op. You can make a copy of this frame to create a new Macro frame)"
        n115 = call <vilib>:"Add State(s) to Queue__JKI_lib_State_Machine.vi"("State(s) in (\"\")"=w320) -> ("States Out"=w319:string)  [unwired: 14 in]
      }
      frame "Macro: Initialize" {
        n116 = call <vilib>:"Add State(s) to Queue__JKI_lib_State_Machine.vi"("State(s) in Front (\"\")"="Data: Initialize\nInitialize Core Data\nEvents: Register\nUI: Initialize\n// UI: Front Panel State >> Open\n\n\nAction: Read Config", "State(s) in (\"\")"=w326) -> ("States Out"=w325:string)  [unwired: 13 in]
      }
      frame "Macro: Update" {
        n117 = call <vilib>:"Add State(s) to Queue__JKI_lib_State_Machine.vi"("State(s) in Front (\"\")"="Action: Write Config", "State(s) in (\"\")"=w332) -> ("States Out"=w331:string)  [unwired: 13 in]
      }
      frame "Macro: Exit" {
        # "Exit Macro\n(This is called once, when the VI exits)"
        n118 = Unbundle By Name(w341) -> ("Core.Close Panel on Exit?"=w340:bool)
        n119 = Select(t="UI: Front Panel State >> Close", s=w340, f="") -> (s? t:f=w337:string)
        n120 = call <vilib>:"Add State(s) to Queue__JKI_lib_State_Machine.vi"("State(s) in Front (\"\")"="Action: Write Config", "State(s) in (\"\")"=w337, "State(s) at Back (\"\")"="Data: Cleanup\nEvents: Unregister\nExit") -> ("States Out"=w335:string)  [unwired: 12 in]
        n121 = call <vilib>:"Add State(s) to Queue__JKI_lib_State_Machine.vi"("State(s) in Front (\"\")"=w335, "State(s) in (\"\")"=w344) -> ("States Out"=w343:string)  [unwired: 13 in]
      }
      frame "---------- Action ----------" {
      }
      frame "Action: Read Config" {
        n122 = call "Read SVW.vi"("GUI in"=w350) -> ("SharedVariableWrapper.lvclass"=w349:refnum<class "SharedVariableWrapper.lvclass">)  [unwired: 10 in]
        n123 = in-place {
          in-place-border: w355 -> [w360]
          in-place-border: [w359] -> w354
          in-place-border: w349 -> [w361]
          n124 = in-place-cluster #1(w353) -> ("settings_name_1"=w358:string)
          n125 = call "Read.vim"("SharedVariableWrapper in"=w361, "name"=w358, "DataType"=T7 {"average size"=0, "open force"=12, "close force"=12, "open settings"={"ACC Steps Per Sec^2"=50, "DEC Steps Per Sec^2"=50, "Min Velosity Step Per Sec"=100, "Max Velosity Step Per Sec"=200, "MicroStep"=16}, "close settings"={"ACC Steps Per Sec^2"=0, "DEC Steps Per Sec^2"=0, "Min Velosity Step Per Sec"=0, "Max Velosity Step Per Sec"=0, "MicroStep"=0}} ("NVM Settings"), "error in (no error)"=w360) -> ("error out"=w359:errorcluster)  [unwired: 5 in, 6 out]
          n126 = in-place-cluster #1("settings_name_1"=w358) -> (w352:T9)
        }
      }
      frame "Action: Write Config" {
        n127 = call "Read ConfigInterface.vi"("GUI in"=w366) -> ()  [unwired: 9 in, 2 out]
        n128 = Unbundle By Name(w364) -> ("amc"=w372:refnum<class "MessageAMC.lvclass">)
        n129 = call "Read SVW.vi"("GUI in"=w366) -> ("SharedVariableWrapper.lvclass"=w375:refnum<class "SharedVariableWrapper.lvclass">)  [unwired: 10 in]
        n130 = call "ReadConfig.vi"("SharedVariableWrapper in"=w375) -> ("config"=w374:T8)  [unwired: 12 in, 2 out]
        n131 = Unbundle By Name(w374) -> ("ip"=w373:string)
        n132 = call "SendNetworkVariant.vi"("reference in"=w372, "receiver process"="STAND", "receiver host"=w373, "receiver port (0)"=u16 54321, "name"="NVM_SETTINGS_1", "data"=variant, "timeout (25000 ms)"=1000, "error in (no error)"=w365) -> ("error out"=w369:errorcluster)  [unwired: 5 in, 2 out]
        n133 = call <vilib>:"Simple Error Handler.vi"("error in (no error)"=w369) -> ("error out"=w363:errorcluster)  [unwired: 4 in, 4 out]
      }
    }
  }
  n134 = call "Read SVW.vi"("GUI in"=w3) -> ("SharedVariableWrapper.lvclass"=w2:refnum<class "SharedVariableWrapper.lvclass">)  [unwired: 10 in]
  n135 = property on="Engine State" class="Ring (strict)"() -> ("Strings []"=w1:string[])  [unwired: 2 in, 2 out]
  n136 = while {
    tunnel: w2 -> [w383]
    tunnel: w1 -> [w378]
    stop <- "stop" stop-if-true
    n137 = stacked-sequence {
      tunnel: w383 -> [w403 w410]
      tunnel: [w401 _] -> w381
      tunnel: [_ w407] -> w382
      tunnel: w378 -> [w388 _]
      frame #0 {
        n138 = call "Read.vim"("SharedVariableWrapper in"=w403, "name"="NVM_DATA_1", "DataType"=T11 {"Engine State"=8, "StateValveModbus"=enum."IDLE", "Alarms"={"OL"=FALSE, "TF"=FALSE, "STL"=FALSE, "OCP"=FALSE, "CPUV"=FALSE, "UVLO"=FALSE, "SPI_ERROR"=FALSE, "Fault"=FALSE, "OL 2"=FALSE, "TF 2"=FALSE, "STL 2"=FALSE, "OCP 2"=FALSE, "CPUV 2"=FALSE, "UVLO 2"=FALSE, "reserved"=TRUE, "InitDone"=TRUE}, "RAW Possition"=124110, "Angele"=0.0, "Step"=0, "Encoder"=0, "Kinematic"={"ACC Steps Per Sec^2"=100, "DEC Steps Per Sec^2"=100, "Min Velosity Step Per Sec"=100, "Max Velosity Step Per Sec"=200, "MicroStep"=16}, "Limits"={"Fault 2 Switch"=FALSE, "Fault 1 Switch"=FALSE, "Center(Home)"=FALSE, "Lower Limit"=FALSE, "Upper Limit"=FALSE}} ("NVM Data")) -> ("data out"=w399:T11, "error out"=w401:errorcluster)  [unwired: 6 in, 5 out]
        n139 = Unbundle By Name(w399) -> ("Alarms"=→"Alarms":T4, "Engine State"=w387:T1, "StateValveModbus"=w389:T12, "Angele"=→"Waveform Chart - Dark 3":dbl, "Step"=→"step":i32, "Encoder"=→"encoder":i32, "Kinematic"=→"Kinematic":T3)  [unwired: 1 out]
        n140 = Index Array(array=w388, index=w387) -> (element=w386:string)
        n141 = Format Into String(format string="DRIVER STATE: %s", w386) -> (resulting string=→"String":string)  [unwired: 2 in, 1 out]
        n142 = Format Into String(format string="VALVE STATE: %s ", w389) -> (resulting string=→"String 2":string)  [unwired: 2 in, 1 out]
      }
      frame #1 {
        n143 = call "Read.vim"("SharedVariableWrapper in"=w410, "name"="DO_ARRAY_OUT", "DataType"=bool[] []) -> ("data out"=w406:bool[], "error out"=w407:errorcluster)  [unwired: 6 in, 5 out]
        n144 = Index Array(array=w406, index=19) -> (element=→"DO 19":bool)
      }
    }
    n145 = Merge Errors(w382, w381) -> (w380:errorcluster)
    n146 = Wait Until Next ms Multiple(millisecond multiple=u32 100) -> ()  [unwired: 1 out]
    n147 = Unbundle By Name(w380) -> ("status"=→"Connect":bool)
  }
  n148 = flat-sequence {
    tunnel: w8 -> [w412]
    frame #0 {
      n149 = local write "stop"(TRUE ("stop")) -> ()
      "error out" <- w412
    }
  }
